vi "viSI16ArrayToByteArray.vi"(1 "input variable":i16[](array[numeric])) -> (0 "output variable":u8[](array[numeric]))   [LabVIEW 2009]
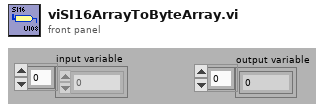
[diagram p1: front panel]
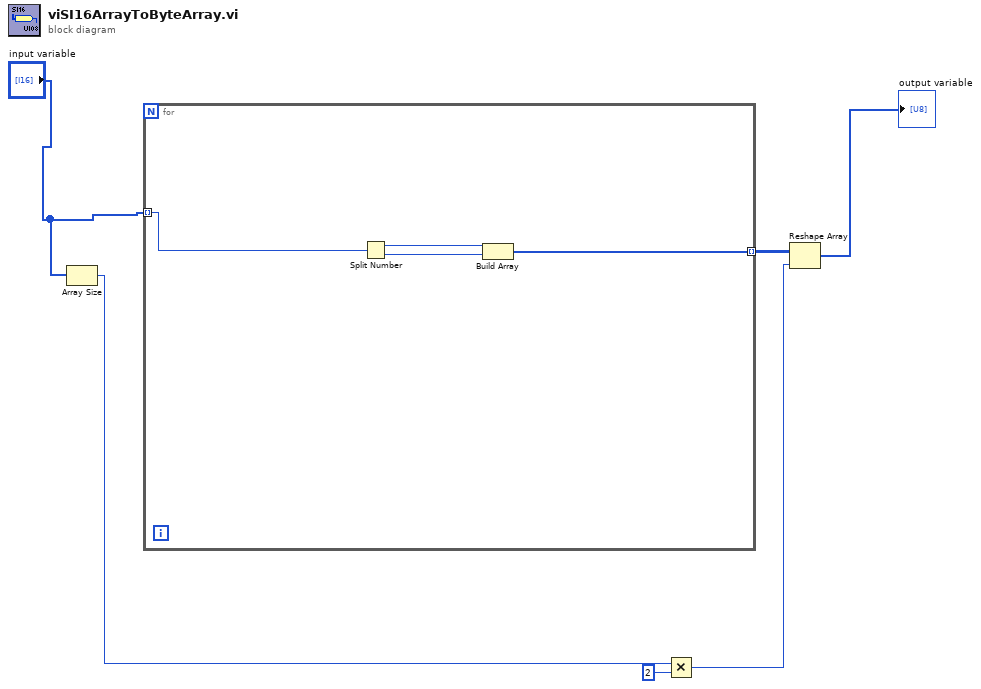
[diagram p0: block diagram]
diagram:
  n1 = Array Size(array="input variable") -> (size(s)=w3:i32)
  n2 = for {
    tunnel: "input variable" -> [w10] mode=indexing
    tunnel: [w7] -> w6 mode=indexing
    n3 = Split Number(x=w10) -> (hi(x)=w9:u8, lo(x)=w8:u8)
    n4 = Build Array(w9, w8) -> (w7:u8[])
  }
  n5 = Multiply(x=w3, y=2) -> (x*y=w2:i32)
  n6 = Reshape Array(w6, w2) -> (→"output variable":u8[])
